vi "PT3_StrsToByteArray.vi"(0 "Length":i32, 1 "String":string, 2 "Length 2":i32, 3 "String 2":string, 4 "Length 3":i32, 5 "String 3":string) -> (16 "Byte Array":u8[](array[numeric]))   [LabVIEW 8.6]
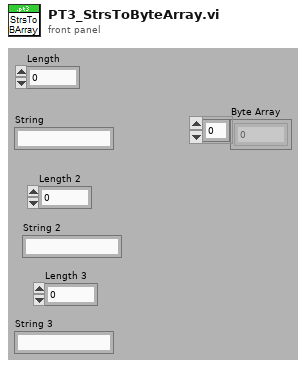
[diagram p1: front panel]
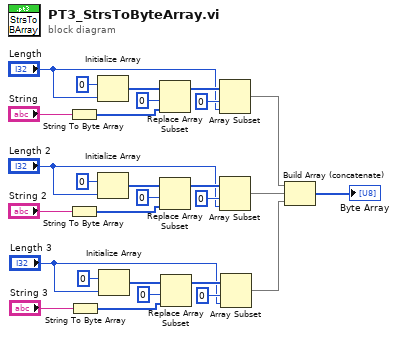
[diagram p0: block diagram]
diagram:
  n1 = String To Byte Array(string="String") -> (unsigned byte array=w27:u8[])
  n2 = String To Byte Array(string="String 2") -> (unsigned byte array=w19:u8[])
  n3 = String To Byte Array(string="String 3") -> (unsigned byte array=w11:u8[])
  n4 = Initialize Array(u8 0 ("element"), "Length") -> (w26:u8[])
  n5 = Initialize Array(u8 0 ("element"), "Length 2") -> (w18:u8[])
  n6 = Initialize Array(u8 0 ("element"), "Length 3") -> (w10:u8[])
  n7 = Replace Array Subset(array=w26, new element=w27, index=0) -> (w23:u8[])
  n8 = Replace Array Subset(array=w18, new element=w19, index=0) -> (w15:u8[])
  n9 = Replace Array Subset(array=w10, new element=w11, index=0) -> (w7:u8[])
  n10 = Array Subset(array=w23, index=0, length="Length") -> (w4:u8[])
  n11 = Array Subset(array=w15, index=0, length="Length 2") -> (w3:u8[])
  n12 = Array Subset(array=w7, index=0, length="Length 3") -> (w2:u8[])
  n13 = Build Array (concatenate)(w4, w3, w2) -> (→"Byte Array":u8[])
